vi "IterateClimber.vi"   [LabVIEW 2015]
uses:
  <vilib>/Rock Robotics/WPI/Utilities/WPI_GetSetVariantRefNum.vi
types:
  T1 = typedef "WPI_JoystickDevRef.ctl" = cluster{"Device":T2}
  T2 = typedef "WPI_JoystickDeviceEnum.ctl" = enum16{"USB 0", "USB 1", "USB 2", "USB 3", "USB 4", "USB 5"}
  T3 = typedef "constants.ctl" = cluster{"motorConstants":cluster{"leftDriveMotor":i32, "rightDriveMotor":i32, "climberAngler":i32, "climberWinch":T4, "shooterTopFlyWheel":T4, "shooterBottomFlyWheel":T4, "climberExtender":i32, "shooterAngler":i32, "shooterIntakeWheel":T4}, "arduinoInputChannel":cluster{"armAngleUp":i32, "intakeWheelSpinIn":i32, "winchUp":i32, "extenderUp":i32}, "driveConstants":cluster{"firstIntervalPercent":dbl, "secondIntervalPercent":dbl, "thirdIntervalPercent":dbl}, "cRioInputChanels":cluster{"photoEye":i32, "limitExtender":i32}, "pneumaticsChannels":cluster{"angleSolenoid":T5}}
  T4 = typedef "FPGA_DIOPWMChannel.ctl" = enum8{"PWM 0", "PWM 1", "PWM 2", "PWM 3", "PWM 4", "PWM 5", "PWM 6", "PWM 7", "PWM 8", "PWM 9", "PWM MXP 0", "PWM MXP 1", "PWM MXP 2", "PWM MXP 3", "PWM MXP 4", "PWM MXP 5", "PWM MXP 6", "PWM MXP 7", "PWM MXP 8", "PWM MXP 9", "Invalid"}
  T5 = typedef "WPI_SolenoidChannel.ctl" = enum8{"Solenoid 0", "Solenoid 1", "Solenoid 2", "Solenoid 3", "Solenoid 4", "Solenoid 5", "Solenoid 6", "Solenoid 7", "Invalid"}
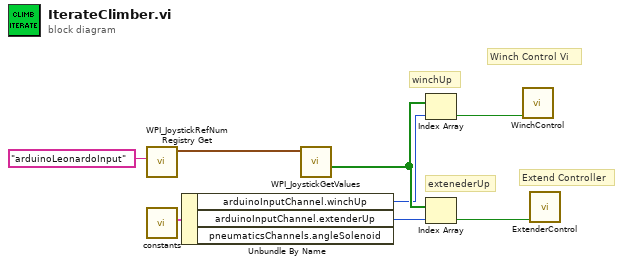
[diagram p0: block diagram]
diagram:
  # "Extend Controller"
  # "Winch Control Vi"
  # "extenederUp"
  # "winchUp"
  n1 = call <vilib>:"WPI_JoystickRefNum Registry Get.vi"("refnum name"="arduinoLeonardoInput") -> ("JoystickDevRef"=w7:T1)  [unwired: 9 in, 1 out]
  n2 = call "constants.vi"() -> (2:w1:T3)  [unwired: 11 in]
  n3 = Unbundle By Name(w1) -> ("arduinoInputChannel.winchUp"=w5:i32, "arduinoInputChannel.extenderUp"=w4:i32)  [unwired: 1 out]
  n4 = call <vilib>:"WPI_JoystickGetValues.vi"("JoystickDevRef"=w7) -> ("Buttons"=w6:bool[])  [unwired: 6 in, 4 out]
  n5 = Index Array(array=w6, index=w5) -> (element=w3:bool)
  n6 = Index Array(array=w6, index=w4) -> (element=w2:bool)
  n7 = call "WinchControl.vi"("arduinoValue"=w3) -> ()  [unwired: 11 in]
  n8 = call "ExtenderControl.vi"("arduinoValue"=w2) -> ()  [unwired: 11 in]
